vi "Initialize.vi"(8 "error in":errorcluster, 10 "shared resources":refnum<class "Shared Resources.lvclass">, 11 "triggers execution unit":refnum<class "Triggers Execution Unit.lvclass">) -> (0 "error out":errorcluster, 3 "triggers execution unit out":refnum<class "Triggers Execution Unit.lvclass">)   [LabVIEW 2020, in "AIM MIL-STD-1553 Engine.lvlib" / "Implementation.lvlib" / "Triggers Execution Unit.lvclass"]
uses:
  Triggers Execution Unit.lvclass
  Interfaces/Shared Resources/Shared Resources.lvclass
  Shared Resources/Shared Resources.lvclass
  Triggers Execution Unit.lvclass/Triggers Execution Unit.ctl
  Execution Unit/Execution Unit.lvclass
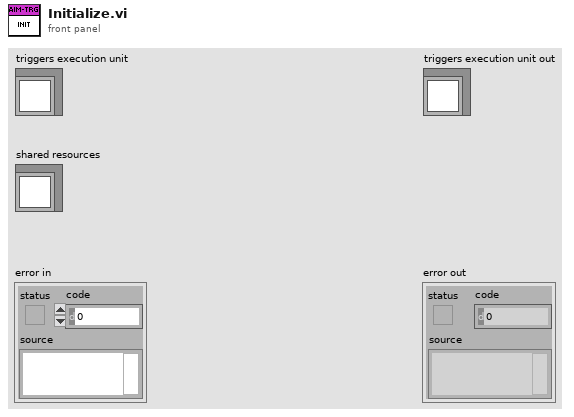
[diagram p1: front panel]
types:
  T1 = typedef "AIM MIL-STD-1553 Engine.lvlib/Implementation.lvlib/Triggers Execution Unit.lvclass/Triggerable Frame.ctl" = cluster{"Acyclic Transfer IDs":u16[], "Acyclic Messages":T2[]}
  T2 = typedef "AIM MIL-STD-1553 Engine.lvlib/Custom Device.lvlib/Compiled Message.ctl" = cluster{"Message Section Handle":T3, "First Parameter Index":i32, "Parameter Channel Handles":T3[], "Direction":T4, "Parameters":T5[], "Receiving RT Address":u8, "Receiving RT Sub-address":u8, "Transmitting RT Address":u8, "Transmitting RT Sub-address":u8, "Word Count":u8, "Buffer Type":enum16{"unknown", "BC Message Buffer", "RT Message Buffer"}, "Buffer ID":u16, "Terminal Type":enum16{"Bus Controller", "Remote Terminal"}, "Timestamp Enabled":bool, "Timestamp Channel Handle":T3}
  T3 = typedef "Custom Device API.lvlib/Custom Device Item Ref.ctl" = u64
  T4 = typedef "Direction.ctl" = enum16{"Rx", "Tx"}
  T5 = typedef "Parameter Definition.ctl" = cluster{"start index":i32, "size (bits)":i32, "encoding":enum16{"BNR", "BCD", "Discrete"}, "signed":bool, "multiplier":dbl, "offset":dbl}
  T6 = typedef "AIM MIL-STD-1553 Engine.lvlib/Custom Device.lvlib/Message Configuration.ctl" = cluster{"Transfer ID":u16, "Transfer Type":enum16{"BC to RT transfer", "RT to BC transfer", "RT to RT transfer"}, "Transmitting RT Address":u8, "Receiving RT Address":u8, "Transmitting RT Sub-address":u8, "Receiving RT Sub-address":u8, "Word Count / Mode Code":u8}
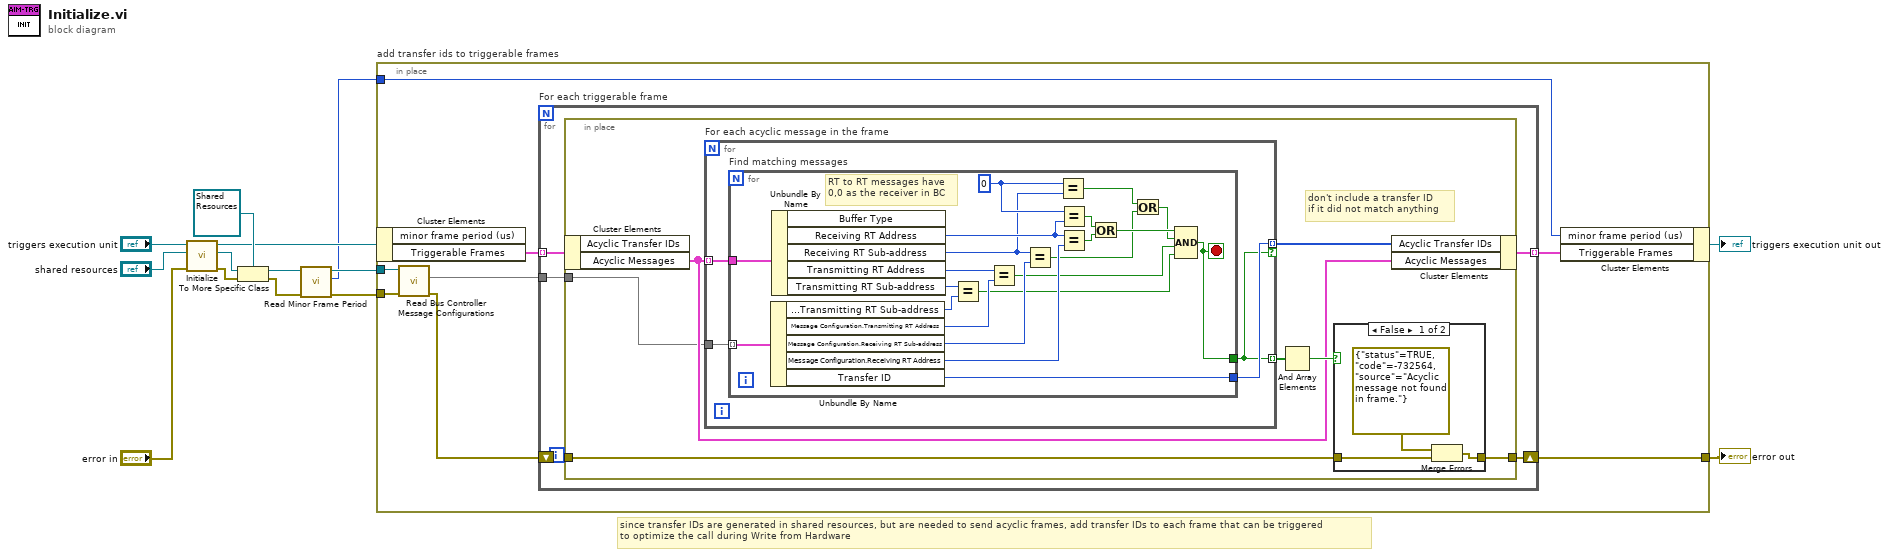
[diagram p0: block diagram]
diagram:
  # "since transfer IDs are generated in shared resources, but are needed to send acyclic frames, add transfer IDs to each frame that can be triggered\nto optimize the call during Write from Hardware"
  n1 = call-parent "Initialize.vi"("error in"="error in", "shared resources"="shared resources", "Execution Unit Implementation in"="triggers execution unit") -> ("error out"=w12:errorcluster, "Execution Unit Implementation out"=w8:refnum<class "Triggers Execution Unit.lvclass">)  [unwired: 7 in]
  n2 = To More Specific Class(target class=refnum<class "Shared Resources.lvclass"> refnum ("Shared Resources in"), reference="shared resources", error in=w12) -> (specific class reference=w4:refnum<class "Shared Resources.lvclass">, error out=w5:errorcluster)
  n3 = call-dynamic "Read Minor Frame Period.vi"("error in (no error)"=w5, "Shared Resources in"=w4) -> ("error out"=w2:errorcluster, "minor frame period (us)"=w1:i32, "Shared Resources out"=w3:refnum<class "Shared Resources.lvclass">)  [unwired: 7 in]
  n4 = in-place "add transfer ids to triggerable frames" {
    in-place-border: w3 -> [w21]
    in-place-border: w2 -> [w17]
    in-place-border: [w15] -> w6
    in-place-border: w1 -> [w14]
    n5 = in-place-cluster #1(w8) -> ("Triggerable Frames"=w19:T1[])  [unwired: 1 out]
    n6 = call-dynamic "Read Bus Controller Message Configurations.vi"("error in"=w17, "shared resources"=w21) -> ("error out"=w16:errorcluster, "messages"=w20:map{u16, T6})  [unwired: 7 in, 1 out]
    n7 = for "For each triggerable frame" {
      tunnel: w20 -> [w26]
      tunnel: w19 -> [w25] mode=indexing
      tunnel: [w24] -> w18 mode=indexing
      shift-right: [w22] -> w15
      shift-left: w16 -> [w23]
      n8 = in-place {
        in-place-border: w26 -> [w27]
        in-place-border: w23 -> [w32]
        in-place-border: [w31] -> w22
        # "don't include a transfer ID\nif it did not match anything"
        n9 = in-place-cluster #2(w25) -> ("Acyclic Messages"=w28:T2[])  [unwired: 1 out]
        n10 = for "For each acyclic message in the frame" {
          tunnel: w27 -> [w41]
          tunnel: w28 -> [w39] mode=indexing
          tunnel: [w40] -> w33 mode=indexing if=w38
          tunnel: [w38] -> w29 mode=indexing
          n11 = for "Find matching messages" {
            tunnel: w39 -> [w62]
            tunnel: w41 -> [w61] mode=indexing
            tunnel: [w52] -> w40
            tunnel: [w51] -> w38
            stop <- w51 stop-if-true
            w50 = 0
            # "RT to RT messages have \n0,0 as the receiver in BC"
            n12 = Unbundle By Name(w61) -> ("Message Configuration.Transmitting RT Sub-address"=w60:u8, "Message Configuration.Transmitting RT Address"=w57:u8, "Message Configuration.Receiving RT Sub-address"=w55:u8, "Message Configuration.Receiving RT Address"=w56:u8, "Transfer ID"=w52:u16)
            n13 = Unbundle By Name(w62) -> ("Receiving RT Address"=w49:u8, "Receiving RT Sub-address"=w48:u8, "Transmitting RT Address"=w58:u8, "Transmitting RT Sub-address"=w59:u8)  [unwired: 1 out]
            n14 = Equal?(x=w59, y=w60) -> (x = y?=w53:bool)
            n15 = Equal?(x=w58, y=w57) -> (x = y?=w54:bool)
            n16 = Equal?(x=w48, y=w55) -> (x = y?=w44:bool)
            n17 = Equal?(x=w50, y=w48) -> (x = y?=w43:bool)
            n18 = Equal?(x=w50, y=w49) -> (x = y?=w46:bool)
            n19 = Equal?(x=w49, y=w56) -> (x = y?=w47:bool)
            n20 = Or(x=w46, y=w47) -> (x .or. y?=w45:bool)
            n21 = Or(x=w43, y=w44) -> (x .or. y?=w42:bool)
            n22 = Compound Arithmetic op=AND(w45, w42, w54, w53) -> (w51:bool)
          }
        }
        n23 = And Array Elements(Boolean array=w29) -> (logical AND=w30:bool)
        n24 = case shown="False" w30 {
          tunnel: w32 -> [w35 w37]
          tunnel: [w34 w37] -> w31
          frame False {
            n25 = Merge Errors(errorcluster {"status"=TRUE, "code"=-732564, "source"="Acyclic message not found in frame."} ("error constant"), w35) -> (w34:errorcluster)
          }
          frame True {
          }
        }
        n26 = in-place-cluster #2("Acyclic Transfer IDs"=w33, "Acyclic Messages"=w28) -> (w24:T1)
      }
    }
    n27 = in-place-cluster #1("minor frame period (us)"=w14, "Triggerable Frames"=w18) -> (→"triggers execution unit out":refnum<class "Triggers Execution Unit.lvclass">)
  }
  "error out" <- w6
